vi "Write Data.vi"(8 "error in (no error)":errorcluster, 10 "Data":refnum<queue>, 11 "HRF_Device in":refnum<class "HRF_Device.lvclass">) -> (0 "error out":errorcluster, 3 "HRF_Device out":refnum<class "HRF_Device.lvclass">)   [LabVIEW 2020]
uses:
  HRF_Device.lvclass
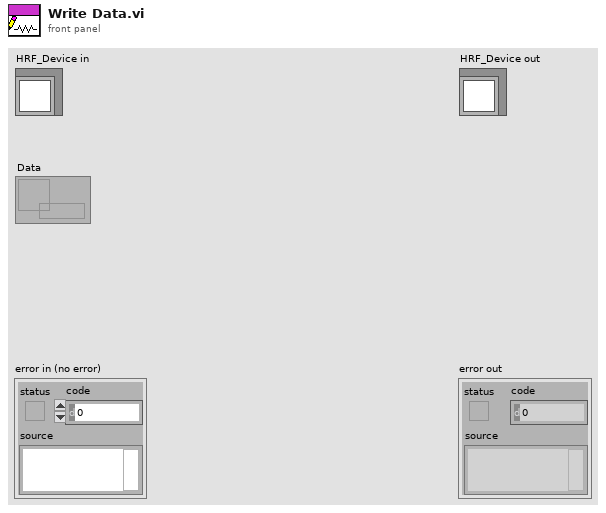
[diagram p1: front panel]
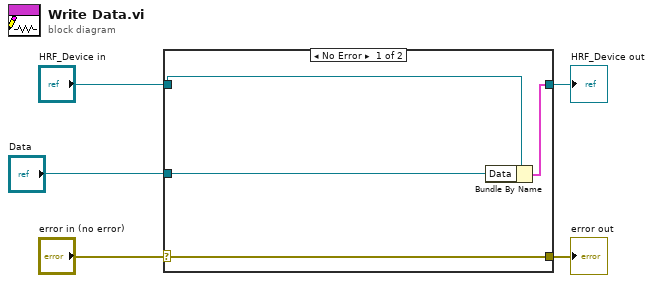
[diagram p0: block diagram]
diagram:
  n1 = case shown="No Error" "error in (no error)" {
    selector: "error in (no error)" -> [w9 w10]
    tunnel: [w9 w10] -> w4
    tunnel: [w6 w11] -> w2
    tunnel: "HRF_Device in" -> [w7 w11]
    tunnel: "Data" -> [w8 _]
    frame No Error {
      n2 = Bundle By Name(cluster=w7, "Data"=w8) -> (w6:cluster{})
    }
    frame Error {
    }
  }
  "error out" <- w4
  "HRF_Device out" <- w2
